vi "Write Teller Metadata.vi"(10 "Teller Metadata":refnum<class "Teller Metadata.lvclass">, 11 "Teller in":refnum<class "Teller.lvclass">) -> (3 "Teller out":refnum<class "Teller.lvclass">)   [LabVIEW 2020, in "jettl.lvlib" / "Teller.lvclass"]
uses:
  Teller.lvclass
  Teller Metadata/Teller Metadata.lvclass
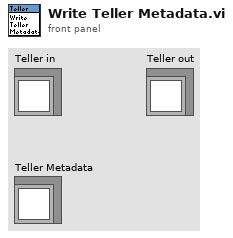
[diagram p1: front panel]
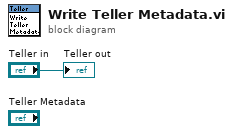
[diagram p0: block diagram]
diagram:
  "Teller out" <- "Teller in"
